vi "Feather Page.vi"() -> ()   [LabVIEW 2020, in "2D Feather.lvclass"]
uses:
  <vilib>/Math Plots/2D Math Plots/2D Feather/2D Feather/2D Feather.lvclass
  <vilib>/Math Plots/2D Math Plots/2D Plot/Action String/2DMathPlot Ctrl Act Queue.ctl
  <vilib>/Math Plots/2D Math Plots/2D Plot/Action String/2DMathPlot Ctrl Act Cluster.ctl
  <vilib>/Math Plots/2D Math Plots/2D Plot/Action String/2DMathPlot State Class.ctl
  <vilib>/Math Plots/2D Math Plots/2D Feather/2D Feather/Typedef/2D Feather Property Cluster.ctl
  <vilib>/Math Plots/2D Math Plots/2D Plot/2D Plot/Typedef/Plot Property Array.ctl
  <vilib>/Math Plots/2D Math Plots/2D Plot/2D Plot/Typedef/Plot Property.ctl
  <vilib>/Math Plots/2D Math Plots/2D Feather/2D Feather/Typedef/2D Feather Property Array.ctl
  <vilib>/Math Plots/2D Math Plots/2D Feather/2D Feather/Typedef/2D Feather Property.ctl
  <vilib>/Math Plots/2D Math Plots/2D Plot/2D Plot/Typedef/Dialog State.ctl
  <vilib>/Math Plots/2D Math Plots/2D Plot/2D Plot/Typedef/Temp Graph State.ctl
  <vilib>/Math Plots/2D Math Plots/2D Plot/2D Plot/Typedef/Temp Graph Property Action.ctl
  <vilib>/Math Plots/2D Math Plots/2D Plot/2D Plot/2D Plot.lvclass
panel:
  in  "Line Color":u32(colorbox) caption="Color"
  out "Feather Property Out":T1={"Plot Property Array"=[{"Bar Plot Style"=0, "DigitalLineStyle"=1, "TransitionLocation"=2, "Transition Type"=0, "Fill To"=-1, "Fill/Pt. Color"=16448250, "Label Style"=3, "Line Style"=0, "Line Width"=0, "Plot Color"=16448250, "Plot Interpolation"=0, "Plot Name"="Plot 0", "Point Style"=1, "Visible?"=TRUE, "XScaleIdx"=0, "YScaleIdx"=0}, {"Bar Plot Style"=0, "DigitalLineStyle"=1, "TransitionLocation"=2, "Transition Type"=0, "Fill To"=-1, "Fill/Pt. Color"=16448250, "Label Style"=3, "Line Style"=0, "Line Width"=0, "Plot Color"=16448250, "Plot Interpolation"=0, "Plot Name"="Plot 1", "Point Style"=1, "Visible?"=TRUE, "XScaleIdx"=0, "YScaleIdx"=0}], "2D Feather Property Array"=[{"Arrow Size"=2.0}, {"Arrow Size"=2.0}]}
  in  "Feather Property In":T1={"Plot Property Array"=[{"Bar Plot Style"=0, "DigitalLineStyle"=1, "TransitionLocation"=2, "Transition Type"=0, "Fill To"=-1, "Fill/Pt. Color"=16448250, "Label Style"=3, "Line Style"=0, "Line Width"=0, "Plot Color"=16448250, "Plot Interpolation"=0, "Plot Name"="Plot 0", "Point Style"=1, "Visible?"=TRUE, "XScaleIdx"=0, "YScaleIdx"=0}, {"Bar Plot Style"=0, "DigitalLineStyle"=1, "TransitionLocation"=2, "Transition Type"=0, "Fill To"=-1, "Fill/Pt. Color"=16448250, "Label Style"=3, "Line Style"=0, "Line Width"=0, "Plot Color"=16448250, "Plot Interpolation"=0, "Plot Name"="Plot 1", "Point Style"=1, "Visible?"=TRUE, "XScaleIdx"=0, "YScaleIdx"=0}], "2D Feather Property Array"=[{"Arrow Size"=2.0}, {"Arrow Size"=2.0}]}
  in  "Event Registration":refnum<event-registration>
  in  "Control Ref Queue":T6
  in  "Arrow Size":dbl=0.001 caption="Size" min=0.001 step=1.0
  in  "Line Width":T7
  in  "Line Style":T8
  in  "Name":string
  in  "Active Plot":i32(ring) items=["Plot 0"]
  # "Line"
  # "Feather"
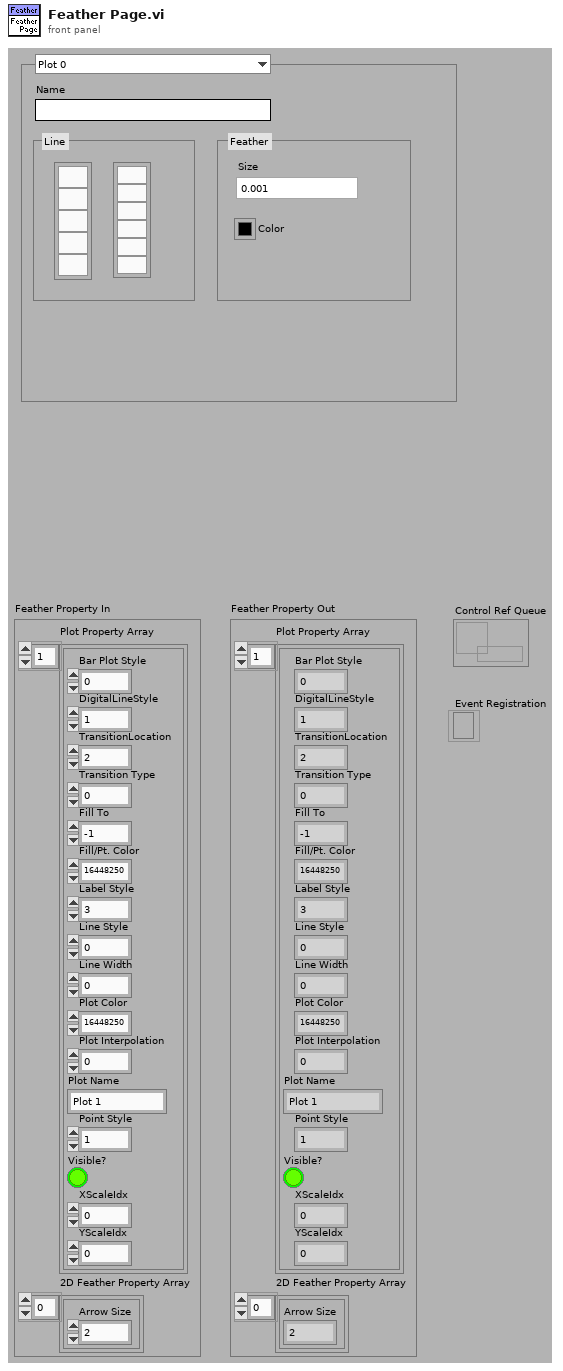
[diagram p1: front panel]
types:
  T1 = typedef "2D Feather.lvclass/2D Feather Property Cluster.ctl" = cluster{"Plot Property Array":T2, "2D Feather Property Array":T4}
  T2 = typedef "2D Plot.lvclass/Plot Property Array.ctl" = T3[]
  T3 = typedef "2D Plot.lvclass/Plot Property.ctl" = cluster{"Bar Plot Style":u8, "DigitalLineStyle":u8, "TransitionLocation":u8, "Transition Type":u8, "Fill To":i16, "Fill/Pt. Color":u32, "Label Style":u8, "Line Style":u8, "Line Width":u8, "Plot Color":u32, "Plot Interpolation":u8, "Plot Name":string, "Point Style":u8, "Visible?":bool, "XScaleIdx":u32, "YScaleIdx":u32}
  T4 = typedef "2D Feather.lvclass/2D Feather Property Array.ctl" = T5[]
  T5 = typedef "2D Feather.lvclass/2D Feather Property.ctl" = cluster{"Arrow Size":dbl}
  T6 = typedef "2DMathPlot Ctrl Act Queue.ctl" = refnum<queue>
  T7 = cluster{"OK Button 2":bool, "OK Button 3":bool, "OK Button 4":bool, "OK Button 5":bool, "OK Button 6":bool, "OK Button 7":bool}
  T8 = cluster{"OK Button":bool, "OK Button 2":bool, "OK Button 3":bool, "OK Button 4":bool, "OK Button 5":bool}
  T9 = typedef "2D Plot.lvclass/Dialog State.ctl" = enum16{"Initialize", "Read Property", "Write Property", "Idle", "Exit"}
  T10 = typedef "2DMathPlot Ctrl Act Cluster.ctl" = cluster{"Plot Area Ref":refnum<vi>, "Z Axis Ref":refnum<vi>, "Legend Ref":refnum<vi>, "XControl Ref":refnum<vi>, "Facade Ref":refnum<vi>, "Display State Change Class":T11}
  T11 = typedef "2DMathPlot State Class.ctl" = enum16{"Update All (Undo)", "Update General", "Update Appearance", "Update Format", "Update Scale", "Update Marker", "Update Cursor", "None"}
  T12 = typedef "2D Plot.lvclass/Temp Graph Property Action.ctl" = enum16{"Appearance Property", "Format Property", "Plots Property", "Scales Property"}
  T13 = typedef "2D Plot.lvclass/Temp Graph State.ctl" = enum16{"Create", "Update Graph", "Update Property Only", "Get Plot Name", "Get Axis Name", "Destory"}
  T14 = cluster{"Bool Array[0]":bool, "Bool Array[1]":bool, "Bool Array[2]":bool, "Bool Array[3]":bool, "Bool Array[4]":bool}
  T15 = cluster{"Bool Array[0]":bool, "Bool Array[1]":bool, "Bool Array[2]":bool, "Bool Array[3]":bool, "Bool Array[4]":bool, "Bool Array[5]":bool}
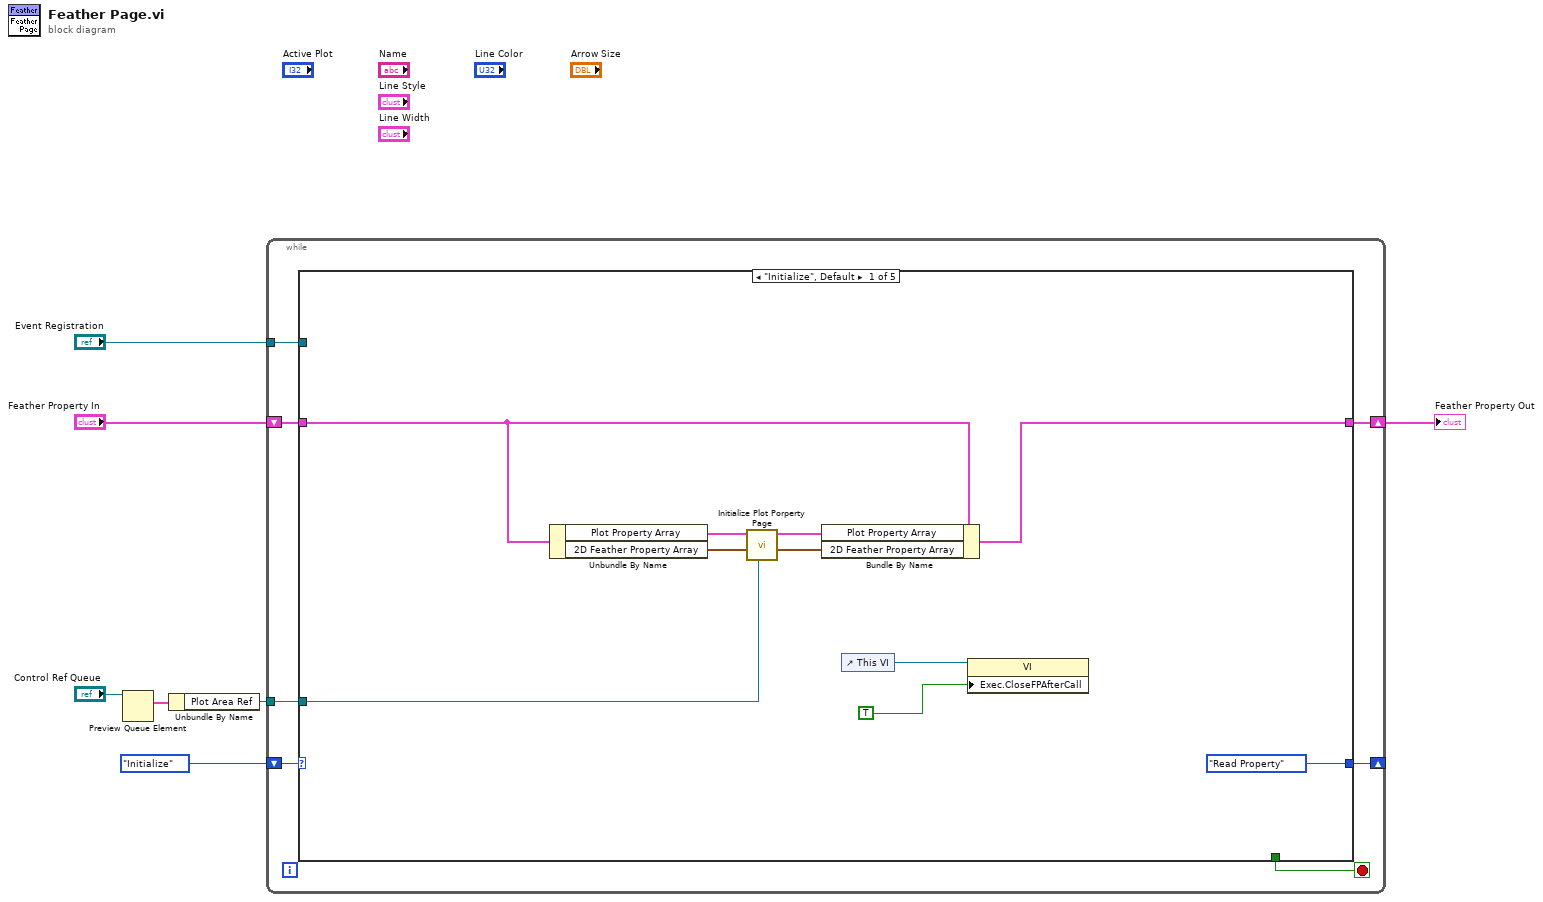
[diagram p0: block diagram]
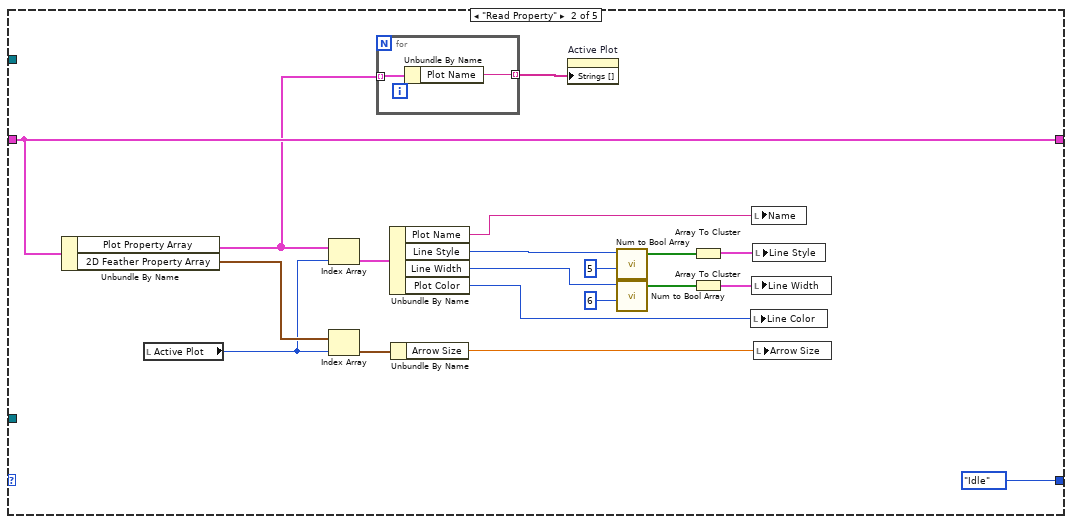
[diagram p2: hidden frame]
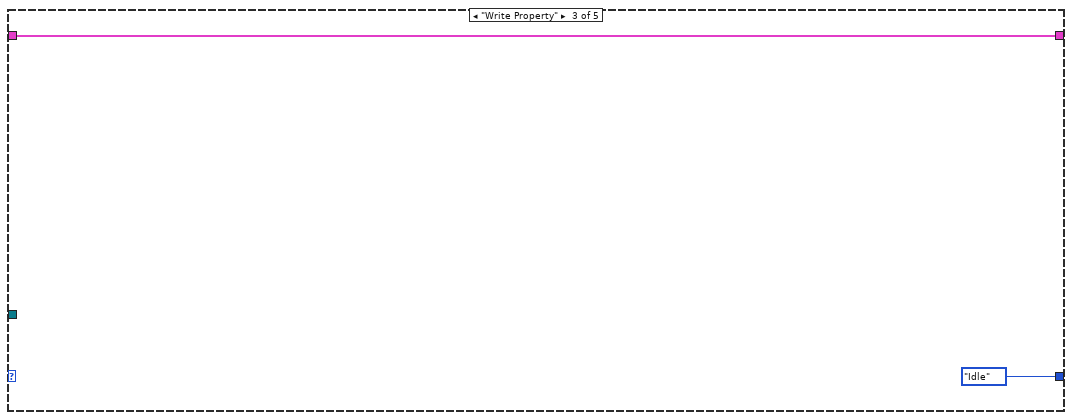
[diagram p3: hidden frame]
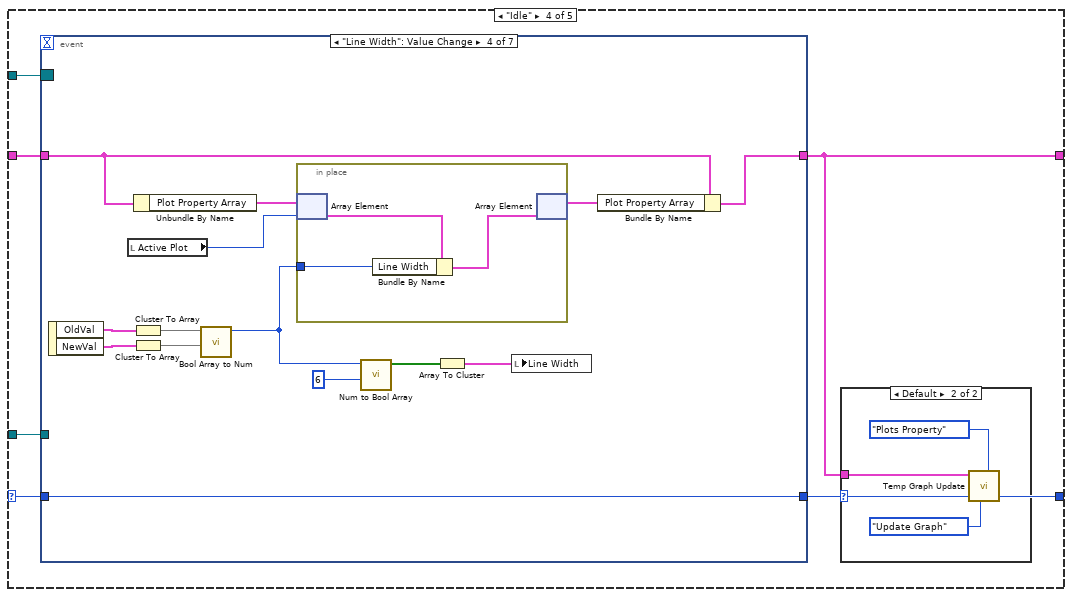
[diagram p4: hidden frame]
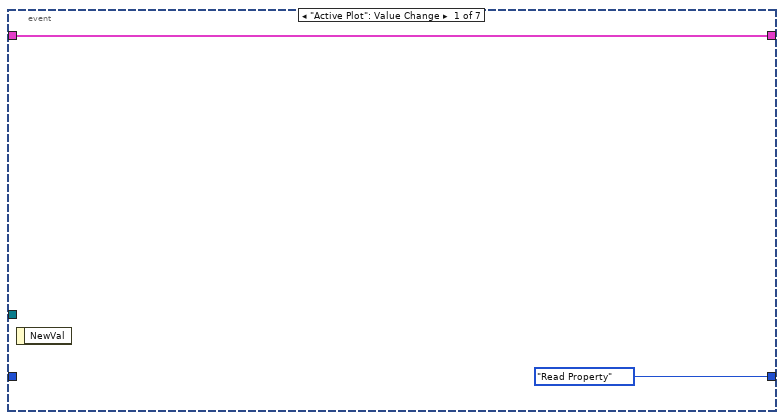
[diagram p6: hidden frame]
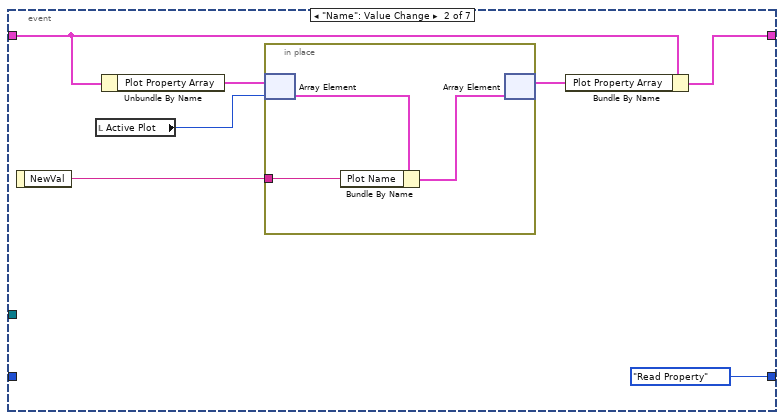
[diagram p7: hidden frame]
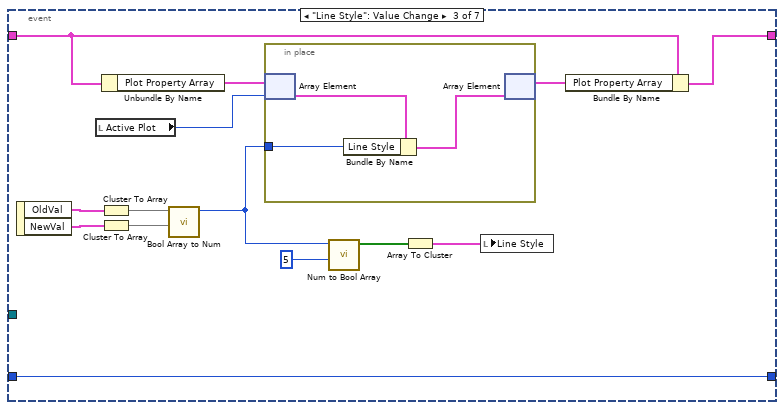
[diagram p8: hidden frame]
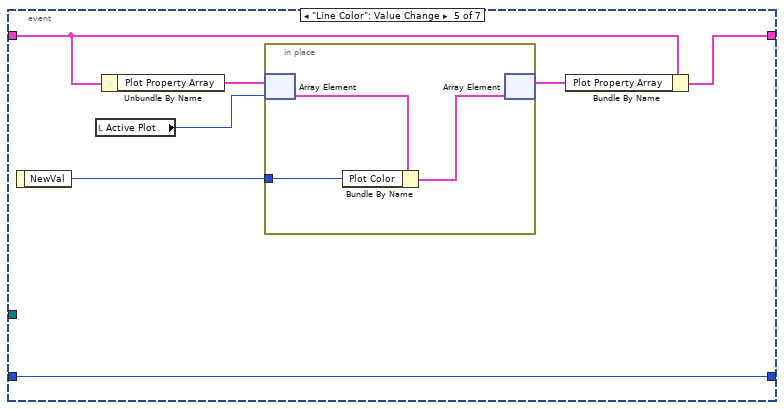
[diagram p9: hidden frame]
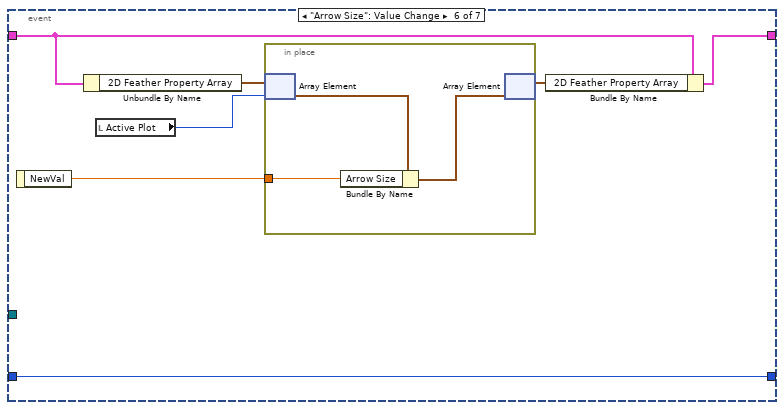
[diagram p10: hidden frame]
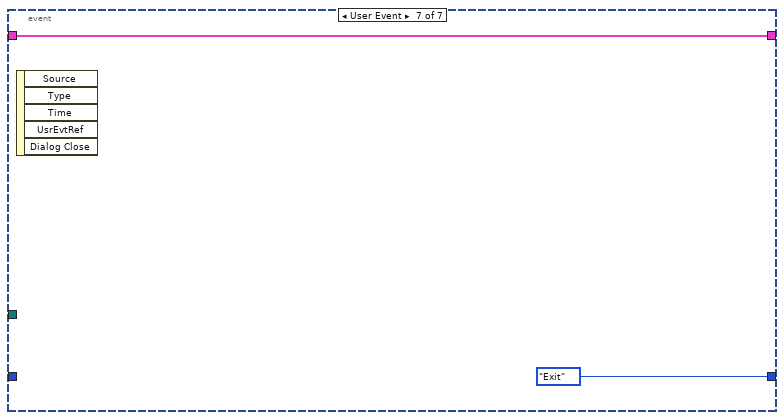
[diagram p11: hidden frame]
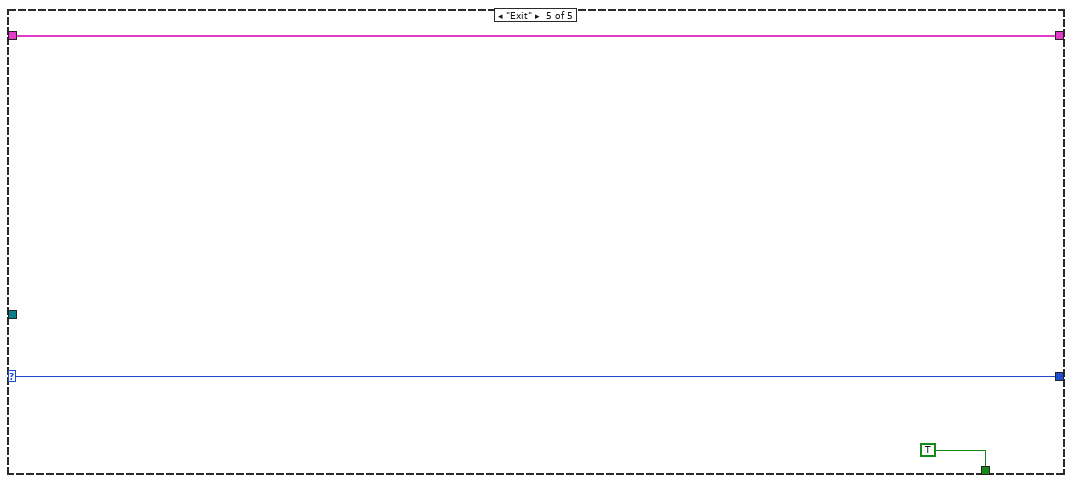
[diagram p12: hidden frame]
diagram:
  n1 = Preview Queue Element(queue="Control Ref Queue") -> (element=w5:T10)  [unwired: 1 in, 4 out]
  n2 = Unbundle By Name(w5) -> ("Plot Area Ref"=w4:refnum<vi>)
  n3 = while {
    tunnel: w4 -> [w13]
    tunnel: "Event Registration" -> [w12]
    shift-right: [w9] -> _
    shift-left: Dialog_State."Initialize" ("Enum") -> [w14]
    shift-right: [w10] -> w1
    shift-left: "Feather Property In" -> [w11]
    stop <- w8 stop-if-true
    n4 = case shown="\"Initialize\", Default" w14 {
      selector: w14 -> [_ _ _ w50 w127]
      tunnel: w13 -> [w15 _ _ w51 _]
      tunnel: w12 -> [_ _ _ w53 _]
      tunnel: w11 -> [w21 w39 w46 w52 w125]
      tunnel: [w20 w39 w46 w49 w125] -> w10
      tunnel: [Dialog_State."Read Property" ("Enum") Dialog_State."Idle" ("Enum") Dialog_State."Idle" ("Enum") w48 w127] -> w9
      tunnel: [_ _ _ _ TRUE] -> w8
      frame "Initialize", Default {
        n5 = Unbundle By Name(w21) -> ("Plot Property Array"=w19:T2, "2D Feather Property Array"=w16:T4)
        n6 = call <vilib>:"Initialize Plot Porperty Page.vi"("Plot Area Ref"=w15, "2D Featherr Array In"=w16, "Plot Property Array In"=w19) -> ("2D Feather Array Out"=w17:T4, "Plot Property Array Out"=w18:T2)  [unwired: 1 in, 6 out]
        n7 = Bundle By Name(cluster=w21, "Plot Property Array"=w18, "2D Feather Property Array"=w17) -> (w20:T1)
        n8 = control-ref of="This VI"() -> (w23:refnum<vi>)
        n9 = property class="VI"(reference=w23, "Exec.CloseFPAfterCall"=TRUE ("Execution:Close After Call")) -> ()  [unwired: 1 in, 2 out]
      }
      frame "Read Property" {
        n10 = Unbundle By Name(w39) -> ("Plot Property Array"=w26:T2, "2D Feather Property Array"=w43:T4)
        n11 = local read "Active Plot"() -> (w42:i32)
        n12 = Index Array(array=w26, index=w42) -> (element=w41:T3)
        n13 = Index Array(array=w43, index=w42) -> (element=w40:T5)
        n14 = for {
          tunnel: w26 -> [w45] mode=indexing
          tunnel: [w44] -> w25 mode=indexing
          n15 = Unbundle By Name(w45) -> ("Plot Name"=w44:string)
        }
        n16 = Unbundle By Name(w41) -> ("Plot Name"=w37:string, "Line Style"=w36:u8, "Line Width"=w29:u8, "Plot Color"=w28:u32)
        n17 = Unbundle By Name(w40) -> ("Arrow Size"=w38:dbl)
        n18 = property on="Active Plot" class="Ring (strict)"("Strings []"=w25) -> ()  [unwired: 2 in, 2 out]
        n19 = call <vilib>:"Num to Bool Array.vi"("Array Size"=5, "Value"=w36) -> ("Bool Array"=w34:bool[])  [unwired: 9 out]
        n20 = call <vilib>:"Num to Bool Array.vi"("Array Size"=6, "Value"=w29) -> ("Bool Array"=w32:bool[])  [unwired: 9 out]
        n21 = Array To Cluster(array=w34) -> (cluster=w33:T14)
        n22 = Array To Cluster(array=w32) -> (cluster=w30:T15)
        n23 = local write "Line Color"(w28) -> ()
        n24 = local write "Name"(w37) -> ()
        n25 = local write "Line Width"(w30) -> ()
        n26 = local write "Line Style"(w33) -> ()
        n27 = local write "Arrow Size"(w38) -> ()
      }
      frame "Write Property" {
      }
      frame "Idle" {
        n28 = event shown="[3] \"Line Width\": Value Change" {
          selector: w53 -> [_ _ _ _ _ _ _]
          dyn-events: _ -> [_ _ _ _ _ _ _]
          timeout: _ -> [_ _ _ _ _ _ _]
          tunnel: w52 -> [w58 w65 w82 w99 w109 w119 w123]
          tunnel: w51 -> [_ _ _ _ _ _ _]
          tunnel: [w58 w64 w81 w98 w108 w118 w123] -> w49
          tunnel: [Dialog_State."Read Property" ("Enum") Dialog_State."Read Property" ("Enum") w69 w86 w104 w114 Dialog_State."Exit" ("Enum")] -> w48
          tunnel: w50 -> [_ _ w69 w86 w104 w114 _]
          event "Active Plot": Value Change {
            n29 = event-data() -> ()  [unwired: 2 out]
          }
          event "Name": Value Change {
            n30 = event-data() -> ("NewVal"=w60:string)  [unwired: 1 out]
            n31 = local read "Active Plot"() -> (w62:i32)
            n32 = Unbundle By Name(w65) -> ("Plot Property Array"=w63:T2)
            n33 = in-place {
              in-place-border: w60 -> [w66]
              n34 = in-place-array #1(w63, w62) -> (w68:T3)
              n35 = Bundle By Name(cluster=w68, "Plot Name"=w66) -> (w67:T3)
              n36 = in-place-array #1(w67) -> (w61:T2)  [unwired: 1 out]
            }
            n37 = Bundle By Name(cluster=w65, "Plot Property Array"=w61) -> (w64:T1)
          }
          event "Line Style": Value Change {
            n38 = event-data() -> ("OldVal"=w73:T8, "NewVal"=w72:T8)  [unwired: 1 out]
            n39 = local read "Active Plot"() -> (w79:i32)
            n40 = Cluster To Array(cluster=w73) -> (array=w75:bool[])
            n41 = Cluster To Array(cluster=w72) -> (array=w74:bool[])
            n42 = Unbundle By Name(w82) -> ("Plot Property Array"=w80:T2)
            n43 = call <vilib>:"Bool Array to Num.vi"("New Bool Array"=w74, "Old Bool Array"=w75) -> ("Value"=w70:u8)  [unwired: 9 out]
            n44 = in-place {
              in-place-border: w70 -> [w83]
              n45 = in-place-array #2(w80, w79) -> (w85:T3)
              n46 = Bundle By Name(cluster=w85, "Line Style"=w83) -> (w84:T3)
              n47 = in-place-array #2(w84) -> (w78:T2)  [unwired: 1 out]
            }
            n48 = call <vilib>:"Num to Bool Array.vi"("Array Size"=5, "Value"=w70) -> ("Bool Array"=w77:bool[])  [unwired: 9 out]
            n49 = Array To Cluster(array=w77) -> (cluster=w71:T14)
            n50 = local write "Line Style"(w71) -> ()
            n51 = Bundle By Name(cluster=w82, "Plot Property Array"=w78) -> (w81:T1)
          }
          event "Line Width": Value Change {
            n52 = event-data() -> ("OldVal"=w90:T7, "NewVal"=w89:T7)  [unwired: 1 out]
            n53 = local read "Active Plot"() -> (w96:i32)
            n54 = Cluster To Array(cluster=w90) -> (array=w92:bool[])
            n55 = Cluster To Array(cluster=w89) -> (array=w91:bool[])
            n56 = Unbundle By Name(w99) -> ("Plot Property Array"=w97:T2)
            n57 = call <vilib>:"Bool Array to Num.vi"("New Bool Array"=w91, "Old Bool Array"=w92) -> ("Value"=w87:u8)  [unwired: 9 out]
            n58 = in-place {
              in-place-border: w87 -> [w100]
              n59 = in-place-array #3(w97, w96) -> (w102:T3)
              n60 = Bundle By Name(cluster=w102, "Line Width"=w100) -> (w101:T3)
              n61 = in-place-array #3(w101) -> (w95:T2)  [unwired: 1 out]
            }
            n62 = call <vilib>:"Num to Bool Array.vi"("Array Size"=6, "Value"=w87) -> ("Bool Array"=w94:bool[])  [unwired: 9 out]
            n63 = Array To Cluster(array=w94) -> (cluster=w88:T15)
            n64 = local write "Line Width"(w88) -> ()
            n65 = Bundle By Name(cluster=w99, "Plot Property Array"=w95) -> (w98:T1)
          }
          event "Line Color": Value Change {
            n66 = event-data() -> ("NewVal"=w103:u32)  [unwired: 1 out]
            n67 = local read "Active Plot"() -> (w106:i32)
            n68 = Unbundle By Name(w109) -> ("Plot Property Array"=w107:T2)
            n69 = in-place {
              in-place-border: w103 -> [w110]
              n70 = in-place-array #4(w107, w106) -> (w112:T3)
              n71 = Bundle By Name(cluster=w112, "Plot Color"=w110) -> (w111:T3)
              n72 = in-place-array #4(w111) -> (w105:T2)  [unwired: 1 out]
            }
            n73 = Bundle By Name(cluster=w109, "Plot Property Array"=w105) -> (w108:T1)
          }
          event "Arrow Size": Value Change {
            n74 = event-data() -> ("NewVal"=w113:dbl)  [unwired: 1 out]
            n75 = Unbundle By Name(w119) -> ("2D Feather Property Array"=w117:T4)
            n76 = local read "Active Plot"() -> (w116:i32)
            n77 = in-place {
              in-place-border: w113 -> [w120]
              n78 = in-place-array #5(w117, w116) -> (w122:T5)
              n79 = Bundle By Name(cluster=w122, "Arrow Size"=w120) -> (w121:T5)
              n80 = in-place-array #5(w121) -> (w115:T4)  [unwired: 1 out]
            }
            n81 = Bundle By Name(cluster=w119, "2D Feather Property Array"=w115) -> (w118:T1)
          }
          event User Event {
            n82 = event-data() -> ()  [unwired: 6 out]
          }
        }
        n83 = case shown="Default" w48 {
          tunnel: w49 -> [_ w54]
          frame "Exit" {
          }
          frame Default {
            n84 = call <vilib>:"Temp Graph Update.vi"("Property Name"=Temp_Graph_Property_Action."Plots Property", "State"=Temp_Graph_State."Update Graph", "Property In"=w54) -> ()  [unwired: 2 in, 7 out]
          }
        }
      }
      frame "Exit" {
      }
    }
  }
  "Feather Property Out" <- w1
